vi "transmitRFID v1.vi"() -> ()   [LabVIEW 2015]
uses:
  Global_bits.vi
  <instrlib>/niUSRP/niUSRP Write Tx Data (CDB).vi
panel:
  out "RN16 array":i32[](array[numeric])
  in  "RFID":bool
  in  "Parameters Query":T1 {"Session" items=["S0", "S1", "S2", "S3"]; "Sel" items=["All", "All2", "~SL", "SL"]; "M" items=["M=1", "M=2", "M=4", "M=8"]}
  out "Bits Graph":i16[](graph)
  out "Waveform Magnitude":dbl[](graph)
  out "Samples":i32
  out "Loop":i32
  in  "Symbol Rate [Hz]":dbl=500000.0 format="%#_13p"
  in  "Parameters Select":T2={"Target"=7, "Action"=0, "MemBank"=1, "truncate"=FALSE} {"MemBank" items=["00 RFU", "01 EPC", "10 TID", "11 User"]; "Action" items=["000", "001", "010", "011", "100", "101", "110", "111"]; "Target" items=["000 Inventoried (S0)", "001 Inventoried (S1)", "010 Inventoried (S2)", "011 Inventoried (S3)", "100 SL", "101 RFU", "110 RFU", "111 RFU"]}
  in  "Parameters Symbols":T3={"Tari"=8e-06, "PW"=0.5, "factor for \"1\" symbol"=0.5, "RTcal"=2.5, "TRcal"=3.0, "Delimiter"=1.25e-05} {"TRcal" min=1.1 max=3.0 step=0.1; "RTcal" min=2.5 max=3.0 step=0.1; "factor for \"1\" symbol" min=0.5 max=1.0 step=0.1; "PW" min=0.265 max=0.525 step=0.001; "Tari" format="%#_3p"}
  out "coerced IQ rate":dbl=100000.0 format="%#_6p"
  out "carrier frequency":dbl=100000.0 format="%#_6p"
  out "coerced gain":dbl format="%#_6f"
  out "error out":errorcluster
  in  "stop":bool
  in  "IQ rate":dbl=2000000.0 format="%#_6p"
  in  "carrier frequency":dbl=920000000.0 format="%#_6p"
  in  "gain":dbl format="%#_6f"
  in  "tx device names":refnum<k15>="192.168.20.13"
  # "Transmit RFID"
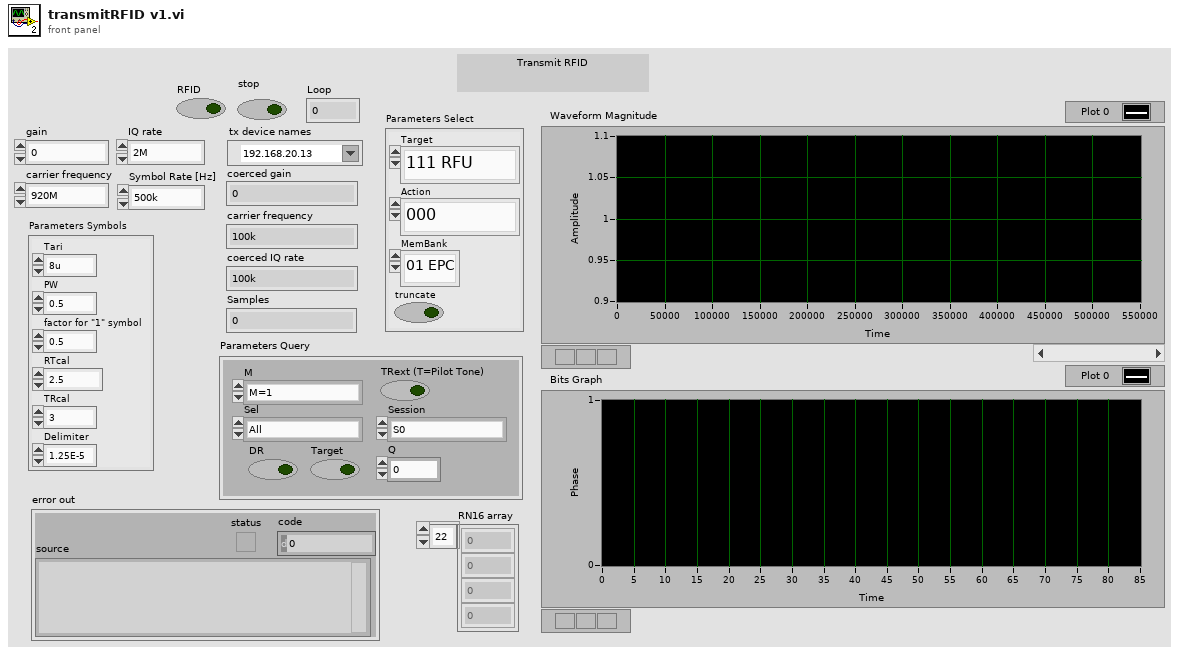
[diagram p1: front panel]
types:
  T1 = cluster{"DR":bool, "M":u16, "TRext (T=Pilot Tone)":bool, "Sel":u16, "Session":u16, "Q":u8, "Target":bool}
  T2 = cluster{"Target":u16, "Action":u16, "MemBank":u16, "truncate":bool}
  T3 = cluster{"Tari":dbl, "PW":dbl, "factor for \"1\" symbol":dbl, "RTcal":dbl, "TRcal":dbl, "Delimiter":dbl}
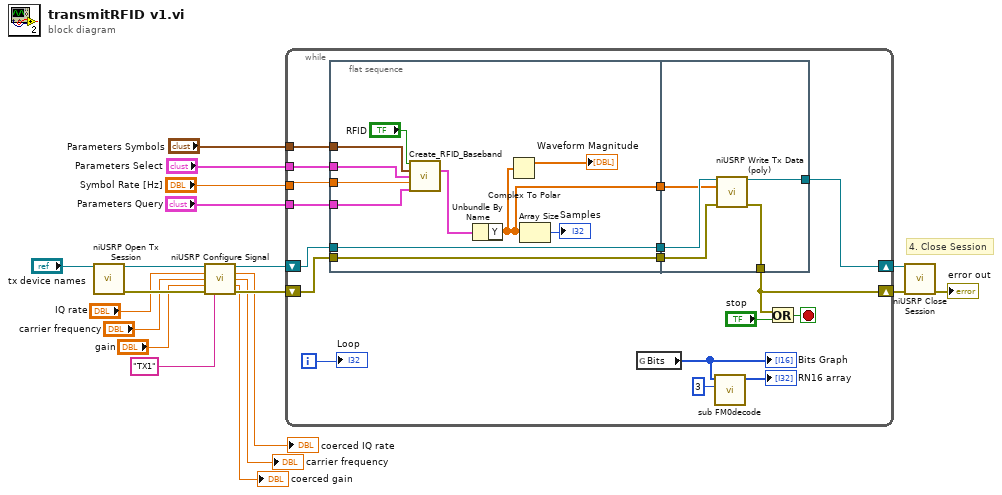
[diagram p0: block diagram]
diagram:
  # "4. Close Session"
  n1 = call <instrlib>:"niUSRP Open Tx Session.vi"("device names"="tx device names") -> ("session handle out"=w4:refnum<k15>, "error out"=w19:errorcluster)  [unwired: 13 in]
  n2 = call <instrlib>:"niUSRP Configure Signal.vi"("session handle"=w4, "IQ rate"="IQ rate", "carrier frequency"="carrier frequency", "gain"="gain", "error in (no error)"=w19, "active antenna"="TX1") -> ("session handle out"=w14:refnum<k15>, "coerced IQ rate"=→"coerced IQ rate":dbl, "coerced carrier frequency"=→"carrier frequency":dbl, "coerced gain"=→"coerced gain":dbl, "error out"=w13:errorcluster)  [unwired: 5 in]
  n3 = while {
    shift-right: [w31] -> w2
    shift-left: w14 -> [w28]
    shift-right: [w30] -> w1
    shift-left: w13 -> [w27]
    tunnel: "Parameters Symbols" -> [w32]
    tunnel: "Parameters Select" -> [w33]
    tunnel: "Symbol Rate [Hz]" -> [w34]
    tunnel: "Parameters Query" -> [w24]
    i -> [w35]
    stop <- w23 stop-if-true
    n4 = flat-sequence {
      tunnel: w34 -> [w46]
      tunnel: w33 -> [w45]
      tunnel: w32 -> [w44]
      tunnel: [w43] -> w29
      tunnel: w28 -> [w43]
      tunnel: w27 -> [w42]
      tunnel: [w42] -> w26
      tunnel: [w38] -> w25
      tunnel: w24 -> [w40]
      tunnel: [w52] -> w31
      tunnel: [w51] -> w30
      tunnel: w29 -> [w50]
      tunnel: w26 -> [w49]
      tunnel: w25 -> [w48]
      frame #0 {
        n5 = call "Create_RFID_Baseband.vi"("RFID"="RFID", "Parameters Symbols"=w44, "Parameters Select"=w45, "Symbol Rate [Hz]"=w46, "Parameters Query"=w40) -> ("complex waveform"=w41:cluster{"t0":dbl, "dt":dbl, "Y":cdb[]})  [unwired: 9 in, 1 out]
        n6 = Unbundle By Name(w41) -> ("Y"=w38:cdb[])
        n7 = Complex To Polar(r * e^(i*theta)=w38) -> (r=→"Waveform Magnitude":dbl[])  [unwired: 1 out]
        n8 = Array Size(array=w38) -> (size(s)=→"Samples":i32)
      }
      frame #1 {
        n9 = call-poly <instrlib>:"niUSRP Write Tx Data (poly).vi"("session handle"=w50, "data"=w48, "error in (no error)"=w49) -> ("session handle out"=w52:refnum<k15>, "error out"=w51:errorcluster)  [unwired: 11 in]
      }
    }
    n10 = global read "Global_bits.vi" "Bits"() -> (w22:i16[])
    "Bits Graph" <- w22
    n11 = call "sub FM0decode.vi"("threshold"=3, "Bit Sequence"=w22) -> ("RN16 array"=→"RN16 array":i32[])  [unwired: 9 in]
    n12 = Or(x=w30, y="stop") -> (x .or. y?=w23:bool)
    "Loop" <- w35
  }
  n13 = call <instrlib>:"niUSRP Close Session.vi"("session handle"=w2, "error in (no error)"=w1) -> ("error out"=→"error out":errorcluster)  [unwired: 13 in]
